vi "PPMS2_Watch.vi"() -> ()   [LabVIEW 2019]
uses:
  <vilib>/lvdsc/historical/Open Trace (Numeric).vi
  <vilib>/lvdsc/historical/Write Trace (Numeric).vi
panel:
  out "last execution time":timestamp=timestamp(3547568694.305166 s since 1904-01-01)
  out "most recent complete file":string="ppms2log_20160529.dat"
  in  "stop":bool
  in  "Pattern to match":string="ppms2log*.dat"
  in  "Folder Path In":path=path "\\\\PPMS2\\Data/PPMS Log"
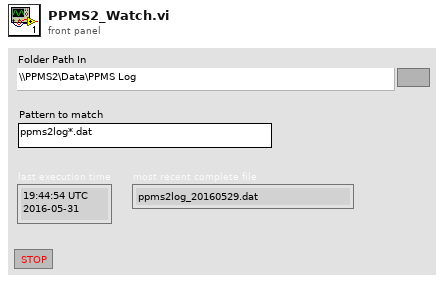
[diagram p1: front panel]
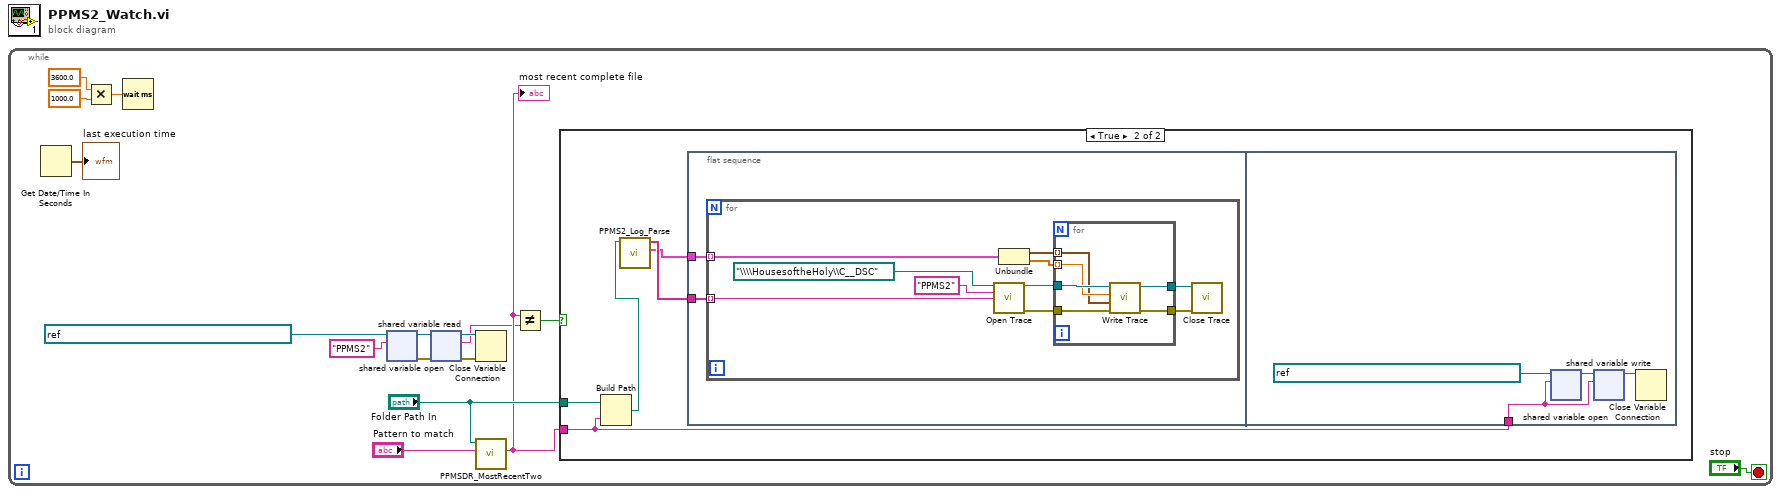
[diagram p0: block diagram]
diagram:
  n1 = while {
    stop <- "stop" stop-if-true
    n2 = Get Date/Time In Seconds() -> (seconds since 1Jan1904=→"last execution time":timestamp)
    n3 = Multiply(x=3600.0, y=1000.0) -> (x*y=w4:dbl)
    n4 = Wait (ms)(milliseconds to wait=w4) -> ()  [unwired: 1 out]
    n5 = shared-variable-open(refnum<k21> "ni.var.psp://localhost/PPMS2/PPMS2 Log" ("shared variable refnum in"), "PPMS2" ("process name")) -> (w11:refnum<k21>, w8:errorcluster)  [unwired: 2 in]
    n6 = shared-variable-read(w11, w8) -> (w10:refnum<k21>, w7:errorcluster, w9:string)  [unwired: 1 out]
    n7 = Close Variable Connection(8:w7, 11:w10) -> ()  [unwired: 1 out]
    n8 = call "PPMSDR_MostRecentTwo.vi"("pattern"="Pattern to match", "directory path"="Folder Path In") -> ("String"=w13:string)  [unwired: 7 in]
    "most recent complete file" <- w13
    n9 = Not Equal?(x=w13, y=w9) -> (x != y?=w6:bool)
    n10 = case shown="True" w6 {
      tunnel: "Folder Path In" -> [_ w21]
      tunnel: w13 -> [_ w20]
      frame False {
      }
      frame True {
        n11 = Build Path(base path=w21, name or relative path=w20) -> (appended path=w17:path)
        n12 = call "PPMS2_Log_Parse.vi"("file path (dialog if empty)"=w17) -> ("XY Graph"=w18:cluster{timestamp[], dbl[]}[], "Array"=w19:string[])  [unwired: 9 in]
        n13 = flat-sequence {
          tunnel: w19 -> [w23]
          tunnel: w18 -> [w22]
          tunnel: w20 -> [w40]
          frame #0 {
            n14 = for {
              tunnel: w23 -> [w27] mode=indexing
              tunnel: w22 -> [w26] mode=indexing
              n15 = call-poly <vilib>:"Open Trace.vi"("database URL"=path "\\\\HousesoftheHoly\\C__DSC", "process name"="PPMS2", "trace name"=w27) -> ("trace reference"=w29:refnum<k1>, "error out"=w28:errorcluster)  [unwired: 10 in, 1 out]
              n16 = Unbundle(w26) -> (w25:timestamp[], w24:dbl[])
              n17 = for {
                tunnel: [w39] -> w31
                tunnel: [w38] -> w30
                tunnel: w29 -> [w37]
                tunnel: w28 -> [w36]
                tunnel: w25 -> [w34] mode=indexing
                tunnel: w24 -> [w35] mode=indexing
                n18 = call-poly <vilib>:"Write Trace.vi"("error in (no error)"=w36, "timestamp (now)"=w34, "value"=w35, "trace ref"=w37) -> ("error out"=w39:errorcluster, "trace ref out"=w38:refnum<k1>)  [unwired: 6 in]
              }
              n19 = call <vilib>:"Close Trace.vi"("error in (no error)"=w31, "trace reference"=w30) -> ()  [unwired: 9 in, 1 out]
            }
          }
          frame #1 {
            n20 = shared-variable-open(refnum<k21> "ni.var.psp://localhost/PPMS2/PPMS2 Log" ("shared variable refnum in"), w40) -> (w42:refnum<k21>)  [unwired: 2 in, 1 out]
            n21 = shared-variable-write(w42, w40) -> (w43:refnum<k21>)  [unwired: 1 in, 1 out]
            n22 = Close Variable Connection(11:w43) -> ()  [unwired: 1 in, 1 out]
          }
        }
      }
    }
  }
